vi "close.vi"(8 "error in":errorcluster, 11 "OPC UA runtime in":refnum<class "OPC UA Client runtime.lvclass">) -> (0 "error out":errorcluster)   [LabVIEW 2014, in "OPC UA Client runtime.lvclass"]
doc: "Close OPC UA Client reference"
uses:
  OPC UA Client runtime.lvclass
  OPC UA Client runtime.lvclass/OPC UA Client runtime.ctl
  <vilib>/OPCUA/NI OPC UA Client.lvlib
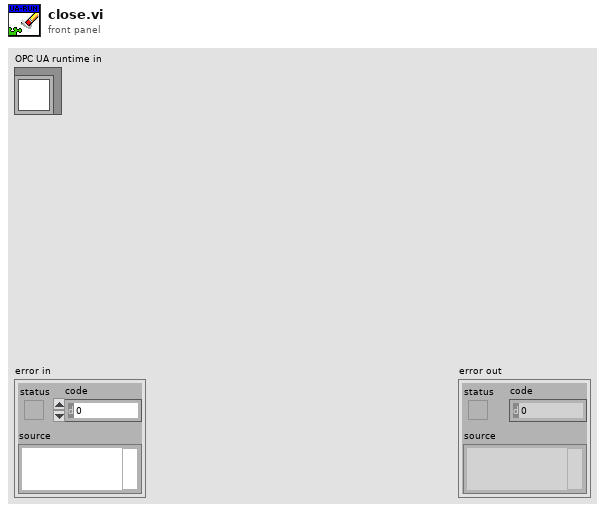
[diagram p1: front panel]
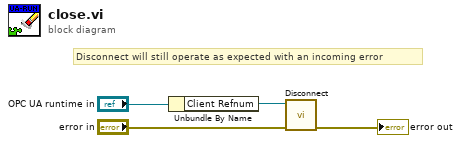
[diagram p0: block diagram]
diagram:
  # "Disconnect will still operate as expected with an incoming error"
  n1 = Unbundle By Name("OPC UA runtime in") -> ("Client Refnum"=w3:refnum<k21>)
  n2 = call <vilib>:"Disconnect.vi"("error in (no error)"="error in", "OPC UA client refnum in"=w3) -> ("error out"=→"error out":errorcluster)  [unwired: 9 in]
